vi "CALC_PAR_DEF_EXT.vi"(0 "VISA IN":refnum<visa-resource-name>, 1 "Measurement Name":string(combo)="S11", 4 "FileName":string, 5 "error in":errorcluster, 7 "Channel":i32=1) -> (14 "VISA Out":refnum<visa-resource-name>, 16 "Meas":string, 18 "FileName":string, 19 "error out":errorcluster)   [LabVIEW 2018, in "PNA-X.lvlib"]
doc: "CALCulate<cnum>:PARameter:DEFine:EXTended <Mname>,<param> \nNote: This command replaces CALC:PAR:DEF as it allows the creating of measurements using \nexternal multiport testsets. \n(Write-only) Creates a measurement but does NOT display it. \nThere is no limit to the number of measurements that can be created. However, there is a limit to the \nnumber of measurements that can be displayed. See Traces, Channels, and Windows on the PNA. \nUse DISP:WIND:STATe to create a window if it doesn't already exist. \nUse DISP:WIND<wnum>:TRAC<tnum>:FEED <Mname> to display the measurement. \nYou must select the measurement (CALC<cnum>:PAR:SEL <mname>) before making additional \nsettings. \nSee Critical Note \nParameters \n1555\n\n<cnum> Channel number of the new measurement. If unspecified, value is set to 1. \n<Mname> (String) Name of the measurement. Any non-empty, unique string, enclosed in \nquotes. \n<param> \n(String ) Measurement Parameter to create. Case sensitive. \nFor S-parameters: \nAny S-parameter available in the PNA \nSingle-digit port numbers CAN be separated by \"_\" (underscore). For \nexample: \"S21\" or \"S2_1\" \nDouble-digit port numbers MUST be separated by underscore. For \nexample: \"S10_1\" \nFor ratioed measurements: \nAny two PNA physical receivers separated by forward slash '/' followed by \ncomma and source port. \nFor example: \"A/R1, 3\" \nLearn more about ratioed measurements \nSee a block diagram showing the receivers in YOUR PNA. \nFor non-ratioed measurements: \nAny PNA physical receiver followed by comma and source port. \nFor example: \"A, 4\" \nLearn more about unratioed measurements. \nSee the block diagram showing the receivers in YOUR PNA. \nWith PNA Rev 6.2, Ratioed and Unratioed measurements can also use logical \nreceiver notation to refer to receivers. This notation makes it easy to refer to \nreceivers with an external test set connected to the PNA. You do not need to \nknow which physical receiver is used for each test port. Learn more. \nFor ADC measurements: \nAny ADC receiver in the PNA followed by a comma, then the source port. \nFor example: \"AI1,2\" indicates the Analog Input1 with source port of 2. \n1556\n\nLearn more about ADC receiver measurements. \nFor Balanced Measurements: \nFirst create an S-parameter measurement, then change the measurement \nusing CALC:FSIM:BAL \"define\" commands. See an example. \nExamples CALC4:PAR:DEF:EXT 'ch4_S33', 'S33' 'Defines an S33 measurement \ncalculate2:parameter:define:extended 'ch1_a', 'b9, 1' 'logical \nreceiver notation for unratioed meas of test port 9 receiver with \nsource port 1. \ncalculate2:parameter:define:extended 'ch1_a', 'b9/a10,1' 'logical \nreceiver notation for ratioed meas of test port 9 receiver divided \nby the reference receiver for port 10 using source port 1 \nQuery Syntax Not Applicable; see Calc:Par:Cat? \nDefault Not Applicable"
uses:
  PNA-X.lvlib
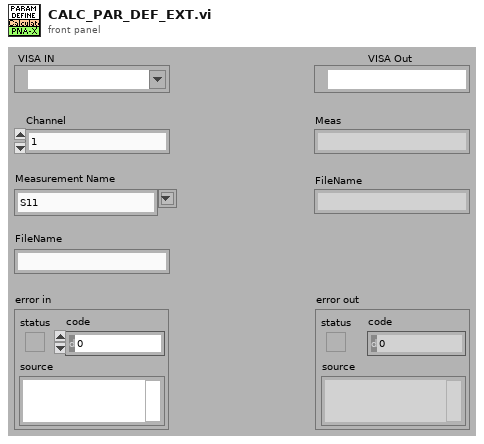
[diagram p1: front panel]
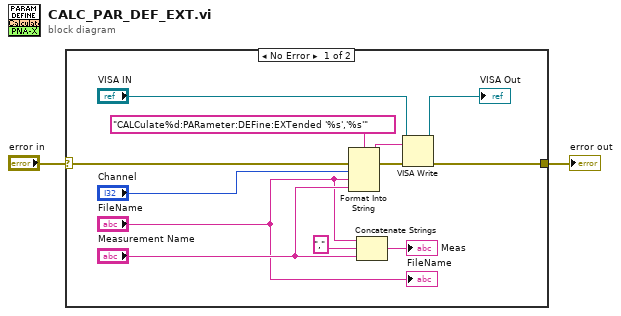
[diagram p0: block diagram]
diagram:
  n1 = case shown="No Error" "error in" {
    selector: "error in" -> [w14 w15]
    tunnel: [w9 w15] -> w1
    frame No Error {
      n2 = Format Into String(format string="CALCulate%d:PARameter:DEFine:EXTended '%s','%s'" ("Cmdline"), error in=w14, "Channel", "FileName", "Measurement Name") -> (resulting string=w12:string, error out=w13:errorcluster)  [unwired: 1 in]
      n3 = Concatenate Strings("FileName", "," ("string"), "Measurement Name") -> (→"Meas":string)
      n4 = VISA Write(VISA resource name="VISA IN", write buffer=w12, error in (no error)=w13) -> (VISA resource name out=→"VISA Out":refnum<visa-resource-name>, error out=w9:errorcluster)  [unwired: 1 out]
      "FileName" <- "FileName"
    }
    frame Error {
    }
  }
  "error out" <- w1
